vi "Update Vehicle Position for Wash Step.vi"(8 "error in (no error)":errorcluster, 10 "Vehicle Pos":u32, 11 "Car Wash Controller Actor in":refnum<class "Car Wash Controller Actor.lvclass">) -> (0 "error out":errorcluster, 3 "Car Wash Controller Actor out":refnum<class "Car Wash Controller Actor.lvclass">)   [LabVIEW 2019]
uses:
  Vehicle Position Simulation/Vehicle Position Simulation Messages/Update Vehicle Position Simulation Msg/Update Vehicle Position Simulation Msg.lvclass
  Car Wash Controller Actor.lvclass
  C:/Program Files (x86)/National Instruments/LabVIEW 2019/vi.lib/ActorFramework/Actor/Actor.lvclass
  <vilib>/ActorFramework/Message Enqueuer/Message Enqueuer.lvclass
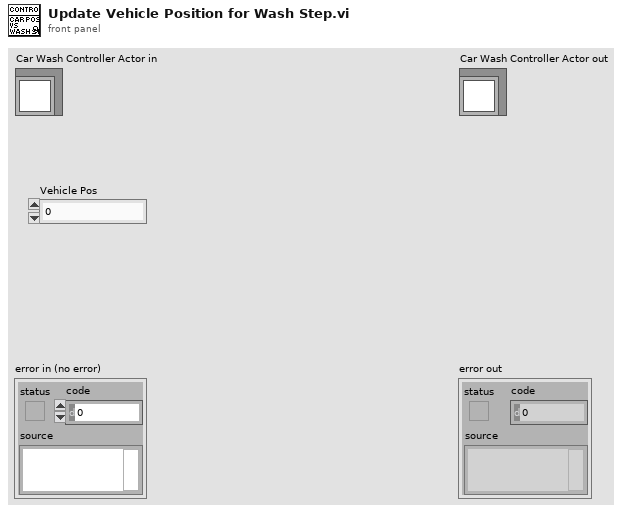
[diagram p1: front panel]
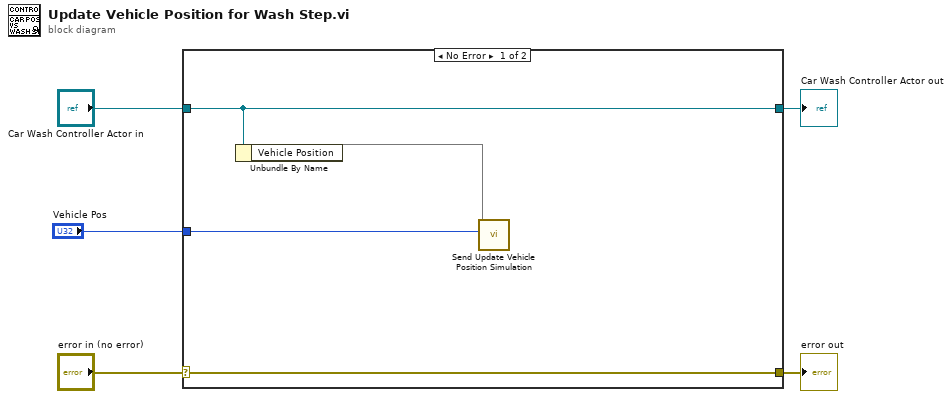
[diagram p0: block diagram]
diagram:
  n1 = case shown="No Error" "error in (no error)" {
    selector: "error in (no error)" -> [w9 w11]
    tunnel: [w9 w11] -> w4
    tunnel: [w8 w10] -> w2
    tunnel: "Car Wash Controller Actor in" -> [w8 w10]
    tunnel: "Vehicle Pos" -> [w6 _]
    frame No Error {
      n2 = Unbundle By Name(w8) -> ("Vehicle Position"=w7)
      n3 = call "Send Update Vehicle Position Simulation.vi"("Vehicle Pos"=w6, "Message Enqueuer"=w7) -> ()  [unwired: 8 in, 2 out]
    }
    frame Error {
    }
  }
  "error out" <- w4
  "Car Wash Controller Actor out" <- w2
